vi "crio_RT_read_serial.vi"() -> ()   [LabVIEW 2019]
panel:
  in  "VISA resource name":refnum<visa-resource-name>
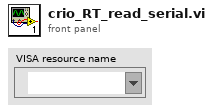
[diagram p1: front panel]
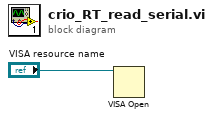
[diagram p0: block diagram]
diagram:
  n1 = VISA Open(VISA resource name="VISA resource name") -> ()  [unwired: 4 in, 2 out]
